vi "Find Nested Libraries.vi"(11 "Library Ref":refnum<vi>) -> (3 "Nested Libraries":T1[](array[typedef]))   [LabVIEW 2021, in "TAF Proj Document Type.lvlib" / "Project Parser.lvlib"]
uses:
  <vilib>/Wovalab/AntiDoc/Document Type/Add-ons/LabVIEW TAF Project/Project Parser/Project Parser.lvlib
  <vilib>/Wovalab/AntiDoc/Document Type/Add-ons/LabVIEW TAF Project/Lib/Nested Lib Info--cluster.ctl
  <vilib>/Wovalab/AntiDoc/Document Type/Add-ons/LabVIEW TAF Project/Lib/Lib.lvclass
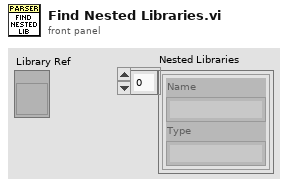
[diagram p1: front panel]
types:
  T1 = typedef "TAF Proj Document Type.lvlib/Lib.lvclass/Nested Lib Info--cluster.ctl" = cluster{"Name":string, "Type":string}
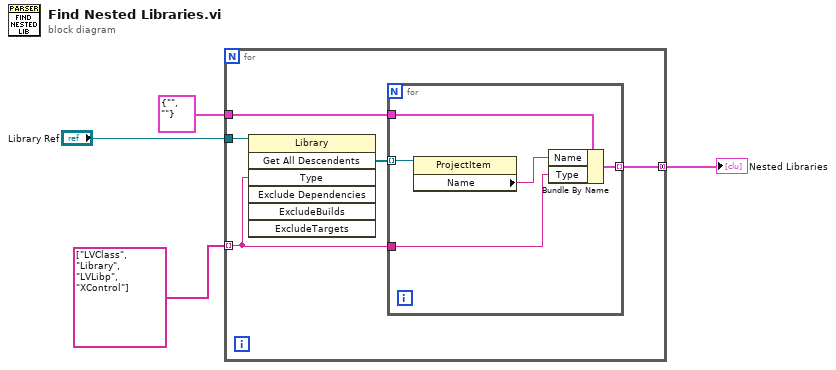
[diagram p0: block diagram]
diagram:
  n1 = for {
    tunnel: "Library Ref" -> [w9]
    tunnel: string[] ["LVClass", "Library", "LVLibp", "XControl"] -> [w6] mode=indexing
    tunnel: T1 {"Name"="", "Type"=""} ("Nested Lib Info") -> [w7]
    tunnel: [w5] -> w1 mode=concatenating
    n2 = invoke class="Library" method="Get All Descendents"(reference=w9, "Type"=w6) -> ("All Descendents"=w8:refnum<vi>[])  [unwired: 5 in, 6 out]
    n3 = for {
      tunnel: w8 -> [w14] mode=indexing
      tunnel: w7 -> [w13]
      tunnel: w6 -> [w11]
      tunnel: [w10] -> w5 mode=indexing
      n4 = property class="ProjectItem"(reference=w14) -> ("Name"=w12:string)  [unwired: 1 in, 2 out]
      n5 = Bundle By Name(cluster=w13, "Name"=w12, "Type"=w11) -> (w10:T1)
    }
  }
  "Nested Libraries" <- w1
